vi "Test_WriteValue_InvalidType_Error.vi"(8 "error in (no error)":errorcluster, 11 "TestCase in":refnum<class "TestTerminalEnabledStateBinding.lvclass">) -> (0 "error out":errorcluster, 3 "TestCase out":refnum<class "TestTerminalEnabledStateBinding.lvclass">)   [LabVIEW 2017, in "TestTerminalEnabledStateBinding.lvclass"]
uses:
  TestTerminalEnabledStateBinding.lvclass
  Source/Concrete/TerminalEnabledStateBinding/TerminalEnabledStateBinding.lvclass
  C:/Git/composed-transport/Source/ITransport/ITransport.lvclass
  Source/ITransport/ITransport.lvclass
panel:
  in  "Numeric":dbl
  out "Return Error":errorcluster
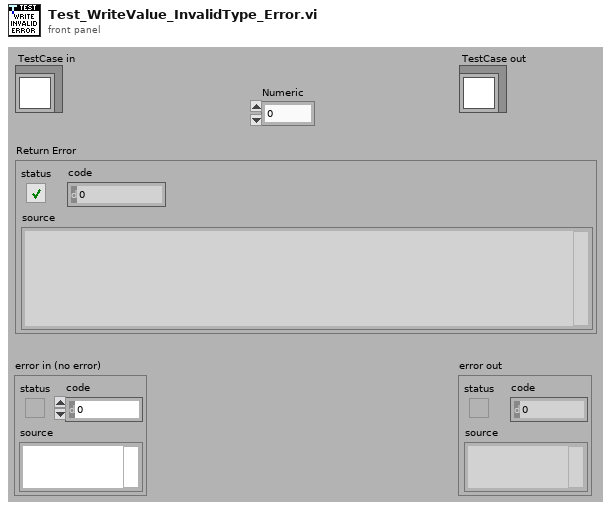
[diagram p1: front panel]
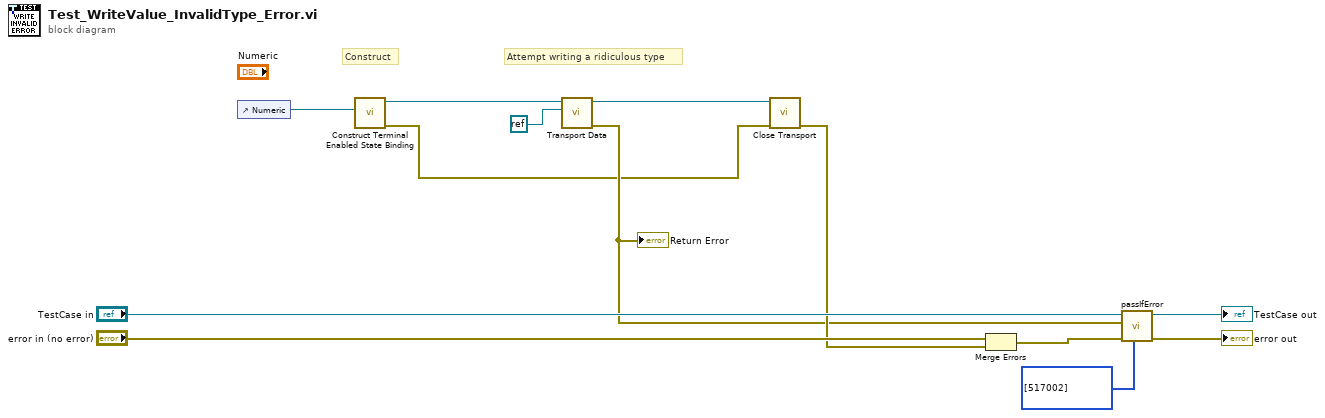
[diagram p0: block diagram]
diagram:
  # "Construct"
  # "Attempt writing a ridiculous type"
  n1 = control-ref of="Numeric"() -> (w2:refnum<vi>)
  n2 = call "Construct Terminal Enabled State Binding.vi"("Control"=w2) -> ("error out"=w1:errorcluster, "TerminalEnabledStateBinding"=w9:refnum<class "TerminalEnabledStateBinding.lvclass">)  [unwired: 9 in]
  n3 = call "Transport Data.vi"("Value"=refnum<k0> refnum, "ITransport in"=w9) -> ("error out"=w5:errorcluster, "ITransport out"=w6:refnum<class "TerminalEnabledStateBinding.lvclass">)  [unwired: 8 in]
  "Return Error" <- w5
  n4 = call-dynamic "Close Transport.vi"("error in (no error)"=w1, "ITransport in"=w6) -> ("error out"=w7:errorcluster)  [unwired: 9 in]
  n5 = Merge Errors("error in (no error)", w7) -> (w8:errorcluster)
  n6 = call-dynamic "passIfError.vi"("passing error codes (default = any error code)"=i32[] [517002], "error in (no error)"=w8, "error"=w5, "TestCase in"="TestCase in") -> ("error out"=→"error out":errorcluster, "TestCase out"=→"TestCase out":refnum<class "TestTerminalEnabledStateBinding.lvclass">)  [unwired: 6 in]
